vi "1D Numeric Integration.vi"(2 "integration method":T1 items=["Trapezoidal Rule", "Simpson's Rule", "Simpson's 3/8 Rule", "Bode Rule"], 3 "dt":dbl=1.0 step=0.001 format="%0.4f", 4 "Input Array":dbl[](array[numeric]) format="%0.2f") -> (0 "error":i32, 1 "result":dbl format="%0.4f")   [LabVIEW 2020, in "NI_AALPro.lvlib"]
doc: "Performs numeric integration on the <B>Input Array</B> using one of four popular numeric integration methods. \n\nWire data to the <B>Input Array</B> input to determine the polymorphic instance to use or manually select the instance."
uses:
  <vilib>/Analysis/NI_AALPro.lvlib
  <vilib>/Analysis/2dsp.llb/Integral Method.ctl
  <resource>/lvanlys.dll
panel:
  # "Numeric Integration"
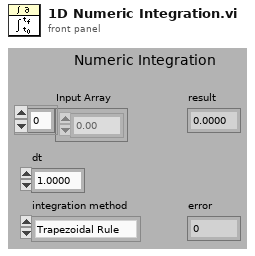
[diagram p1: front panel]
types:
  T1 = typedef "NI_AALPro.lvlib/Integral Method.ctl" = i32
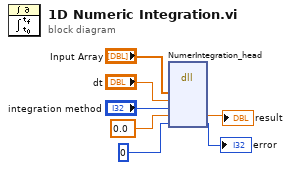
[diagram p0: block diagram]
diagram:
  n1 = dll-call lib="e:/builds/penguin/labview/branches/2020/dev/dist/resource/lvanlys.*" fn="NumerIntegration_head"("Input Array"="Input Array", "dt"="dt", "integration method"="integration method", "output param"=0.0, "output param"=0) -> ("output param"=→"result":dbl, "output param"=→"error":i32)  [unwired: 6 in, 3 out]
